vi "OffsetCalculator.vi"(2 "Array":dbl[][](array[numeric]), 3 "error in (no error)":errorcluster, 4 "Resolution X":u16, 8 "Resolution Y":u16) -> (7 "ProjectedPosition":cluster{dbl, dbl}, 9 "Distances (Inches)":dbl)   [LabVIEW 2012]
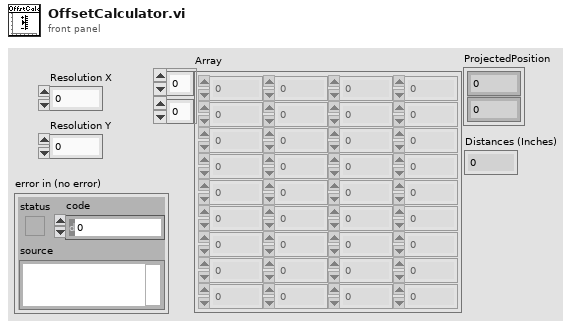
[diagram p1: front panel]
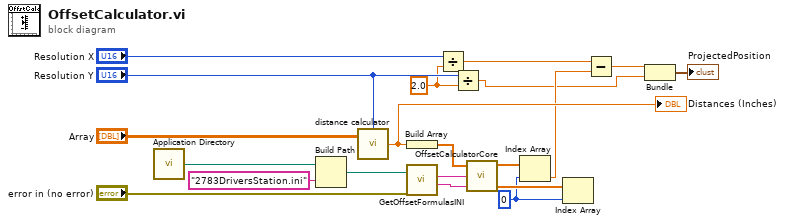
[diagram p0: block diagram]
diagram:
  w5 = 0
  w9 = 2.0 ("y")
  n1 = call <vilib>:"Application Directory.vi"() -> ("Application Directory"=w16:path)
  n2 = Build Path(base path=w16, name or relative path="2783DriversStation.ini") -> (appended path=w14:path)
  n3 = call "distance calculator.vi"("Resolution Y"="Resolution Y", "Array"="Array") -> ("Distances (Inches)"=w18:dbl)  [unwired: 1 in]
  "Distances (Inches)" <- w18
  n4 = Build Array(w18) -> (w17:dbl[])
  n5 = call "GetOffsetFormulasINI.vi"("configuration file path"=w14, "error in (no error)"="error in (no error)") -> ("HorzOffsetFormula"=w19:string, "VertOffsetFormula"=w20:string)  [unwired: 2 out]
  n6 = Divide(x="Resolution X", y=w9) -> (x/y=w8:dbl)
  n7 = Divide(x="Resolution Y", y=w9) -> (x/y=w1:dbl)
  n8 = call "OffsetCalculatorCore.vi"("VertOffsetFormula"=w20, "HorzOffsetFormula"=w19, "Distance"=w17) -> ("VertOffset"=w6:dbl[], "HorzOffset"=w7:dbl[])
  n9 = Index Array(array=w7, index=w5) -> (element=w4:dbl)
  n10 = Index Array(array=w6, index=w5) -> ()  [unwired: 1 out]
  n11 = Subtract(x=w8, y=w4) -> (x-y=w3:dbl)
  n12 = Bundle(w3, w1) -> (→"ProjectedPosition":cluster{dbl, dbl})  [unwired: 1 in]
